vi "Get System Name.vi"(8 "error in (no error)":errorcluster, 11 "Motors in":refnum<class "Motors.lvclass">) -> (0 "error out":errorcluster, 2 "System Name":string, 3 "Motors out":refnum<class "Motors.lvclass">)   [LabVIEW 2014, in "Motors.lvlib" / "Motors.lvclass"]
uses:
  Motors.lvclass
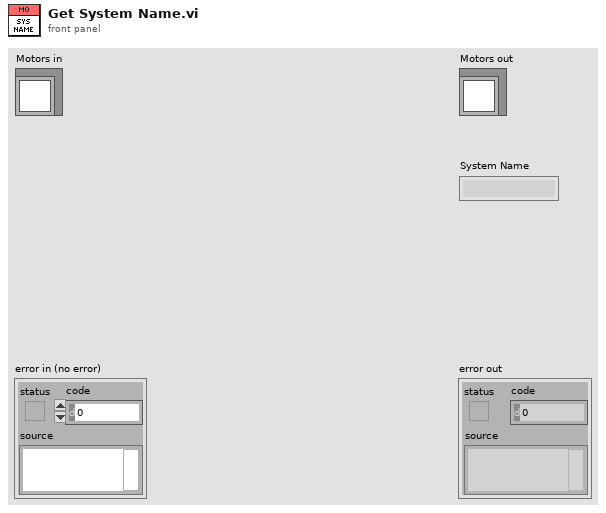
[diagram p1: front panel]
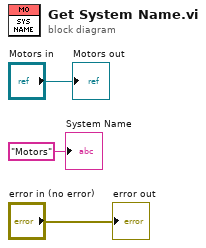
[diagram p0: block diagram]
diagram:
  "error out" <- "error in (no error)"
  "Motors out" <- "Motors in"
  "System Name" <- "Motors" ("System Name")
